vi "SalcompMESSaveResultXML).vi"(10 "XmlFileContent":string) -> (2 "SaveResult":bool)   [LabVIEW 2018]
uses:
  CMESAPI.dll
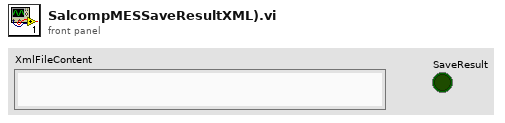
[diagram p1: front panel]
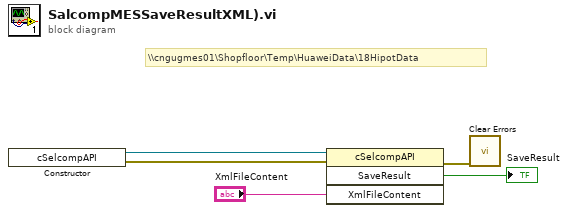
[diagram p0: block diagram]
diagram:
  # "\\\\cngugmes01\\Shopfloor\\Temp\\HuaweiData\\18HipotData"
  n1 = constructor class="cSelcompAPI"() -> (reference out=w5:refnum<k24>, error out=w4:errorcluster)  [unwired: 3 in, 1 out]
  n2 = invoke class="cSelcompAPI" method="SaveResult"(reference=w5, error in=w4, "XmlFileContent"="XmlFileContent") -> (error out=w1:errorcluster, "SaveResult"=→"SaveResult":bool)  [unwired: 1 in, 2 out]
  n3 = call <vilib>:"Clear Errors.vi"("error in (no error)"=w1) -> ()  [unwired: 5 in, 2 out]
